vi "day 3 task 1.vi"() -> ()   [LabVIEW 2019]
uses:
  8b16236f-c8de-4b08-a6c4-6a4b4e7bf06e.vi
panel:
  out "sum (answer)":u64
  out "priorities of items":u8[][](array[numeric])
  out "error log":string[](array[string])
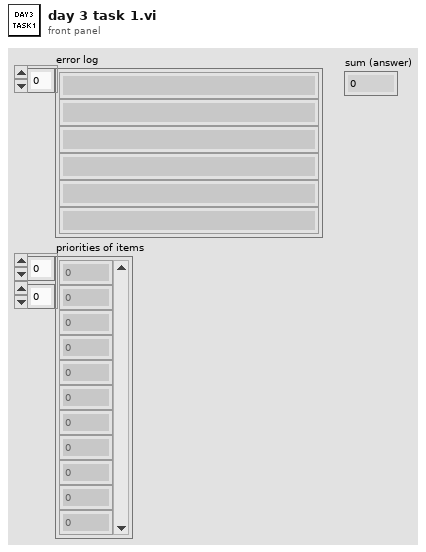
[diagram p1: front panel]
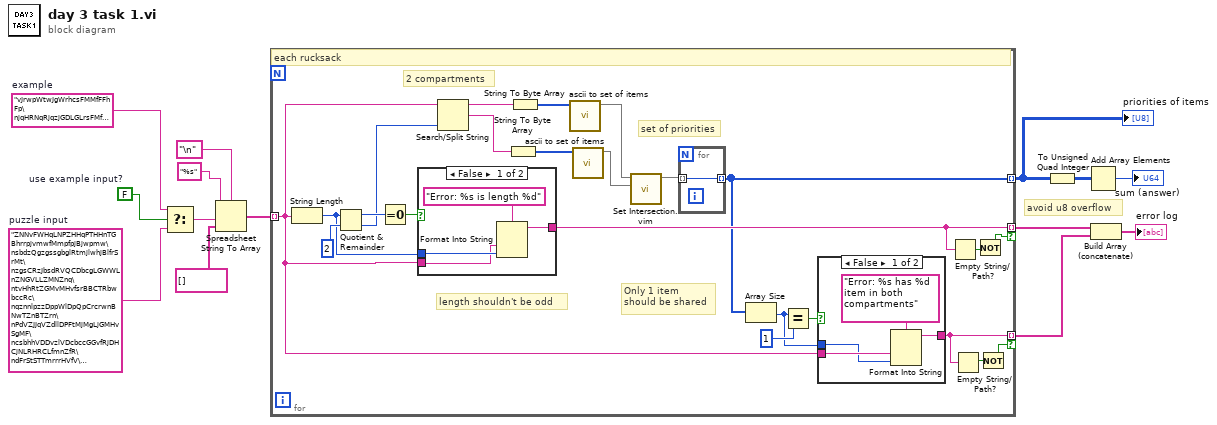
[diagram p0: block diagram]
diagram:
  w9 = FALSE  # use example input?
  w10 = "ZNNvFWHqLNPZHHqPTHHnTGBhrrpjvmwfMmpfpjBjwpmw\nsbdzQgzgssgbglRtmjlwhjBlfrSrMt\nzgsCRzJbsdRVQCDbcgLGWWLnZNGVLLZMNZnq\ntvHhRtZGMvMHvfsrBBCTRbwbccRc\nqznnlpzzDppWlDpQpCrcrwnBNwTZnBTZrn\nPdVZJJqVZdllDPFtMjMgLjGMHvSgMF\ncsbhhVDDvzlVDcbccGGvfRjDHCjNLRHRCLfmnZfR\ndFrStSTTmrrrHVfV\nMMgQMMTMVTdgWtwTPwSgWSgGbbppJzlplvhBlPbzhlhbzG\nFDJSTtSGhpPFDmFTZDpTFPmCBBrHqsCBhgBlqqrqrlRrHH\ndQwMtfdzVwWfwctwnfnQCHllzRrsNzrrgNlCgqsr\nfLfQnVjfwQfMdfvfnVvWDvtJPFGDpvZGbZpmbSPP\nTzzCrJcDrTDdLDCJDvGNPCFqlZWlvNvWpq\nRRHfjsQBFsjgjBQsWqGpNvZQqQlPPQPN\nVnHBnRVssnnjsSfBwbMSrrbTwJTcwSDF\nHJCgHCCFFFVGJWTlbqDdlqTDDpgl\ncZccSmLrfZcrmmzSQftdpDtTHdbQ..."  # puzzle input
  w11 = "vJrwpWtwJgWrhcsFMMfFFhFp\njqHRNqRjqzjGDLGLrsFMfFZSrLrFZsSL\nPmmdzqPrVvPwwTWBwg\nwMqvLMZHhHMvwLHjbvcjnnSBnvTQFn\nttgJtRGJQctTZtZT\nCrZsJsPPZsGzwwsLwLmpwMDw"  # example
  # "avoid u8 overflow"
  n1 = Select(t=w11, s=w9, f=w10) -> (s? t:f=w8:string)
  n2 = Spreadsheet String To Array(delimiter (Tab)="\n", format string="%s", spreadsheet string=w8, array type (2D Dbl)=string[] []) -> (array=w7:string[])
  n3 = for {
    tunnel: w7 -> [w27] mode=indexing
    tunnel: [w17] -> w2 mode=indexing
    tunnel: [w25] -> w6 mode=indexing if=w24
    tunnel: [w22] -> w5 mode=indexing if=w20
    # "2 compartments"
    # "length shouldn't be odd"
    # "Only 1 item\nshould be shared"
    # "set of priorities"
    # "each rucksack"
    n4 = String Length(string=w27) -> (length=w34:i32)
    n5 = Quotient & Remainder(x=w34, y=2) -> (x-y*floor(x/y)=w36:i32, floor(x/y)=w33:i32)
    n6 = Equal To 0?(x=w36) -> (x = 0?=w35:bool)
    n7 = case shown="False" w35 {
      tunnel: w34 -> [w45 _]
      tunnel: w27 -> [w44 _]
      tunnel: [w43 _] -> w22
      frame False {
        n8 = Format Into String(format string="Error: %s is length %d", w44, w45) -> (resulting string=w43:string)  [unwired: 2 in, 1 out]
      }
      frame True {
      }
    }
    n9 = Search/Split String(string=w27, offset (0)=w33) -> (substring before match=w32:string, match + rest of string=w18:string)  [unwired: 1 in, 1 out]
    n10 = String To Byte Array(string=w18) -> (unsigned byte array=w16:u8[])
    n11 = String To Byte Array(string=w32) -> (unsigned byte array=w15:u8[])
    n12 = call "ascii to set of items.vi"("ascii bytes"=w15) -> ("set out"=w31:set{u8})  [unwired: 10 in]
    n13 = call "ascii to set of items.vi"("ascii bytes"=w16) -> ("set out"=w30:set{u8})  [unwired: 10 in]
    n14 = call "Set Intersection.vim"("set 2"=w30, "set 1"=w31) -> ("intersection"=w29:set{u8})  [unwired: 9 in]
    n15 = for {
      tunnel: [w42] -> w17 mode=indexing
      tunnel: w29 -> [w42] mode=indexing
    }
    n16 = Array Size(array=w17) -> (size(s)=w19:i32)
    n17 = Equal?(x=w19, y=1) -> (x = y?=w26:bool)
    n18 = case shown="False" w26 {
      tunnel: w27 -> [w40 _]
      tunnel: [w39 _] -> w25
      tunnel: w19 -> [w38 _]
      frame False {
        n19 = Format Into String(format string="Error: %s has %d item in both compartments", w40, w38) -> (resulting string=w39:string)  [unwired: 2 in, 1 out]
      }
      frame True {
      }
    }
    n20 = Empty String/Path?(string/path=w22) -> (empty?=w21:bool)
    n21 = Empty String/Path?(string/path=w25) -> (empty?=w23:bool)
    n22 = Not(x=w21) -> (.not. x?=w20:bool)
    n23 = Not(x=w23) -> (.not. x?=w24:bool)
  }
  "priorities of items" <- w2
  n24 = To Unsigned Quad Integer(1:w2) -> (0:w3:u64[][])
  n25 = Add Array Elements(numeric array=w3) -> (sum=→"sum (answer)":u64)
  n26 = Build Array (concatenate)(w5, w6) -> (→"error log":string[])
